vi "validate configuration.vi"(8 "error in":errorcluster, 11 "Profibus Module configuration in":refnum<class "Profibus Module configuration.lvclass">) -> (0 "error out":errorcluster, 3 "Profibus Module configuration out":refnum<class "Profibus Module configuration.lvclass">)   [LabVIEW 2013, in "Profibus Module configuration.lvclass"]
doc: "This function performs validation of the configuration. This function should be safe to call at any point and should not rely on anything in the runtime environment."
uses:
  Profibus Module configuration.lvclass
  <vilib>/NI/Tag Bus Module Framework/module configuration/TBM module configuration.lvclass
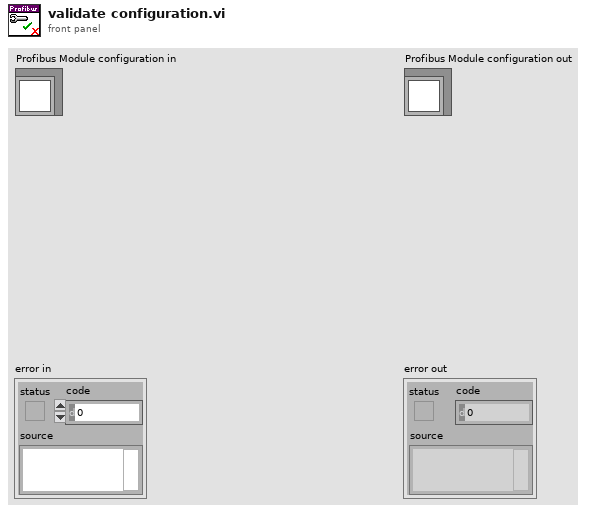
[diagram p1: front panel]
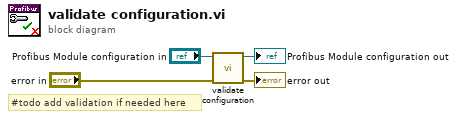
[diagram p0: block diagram]
diagram:
  # "#todo add validation if needed here"
  n1 = call-parent "validate configuration.vi"("error in"="error in", "configuration in"="Profibus Module configuration in") -> ("error out"=→"error out":errorcluster, "configuration out"=→"Profibus Module configuration out":refnum<class "Profibus Module configuration.lvclass">)  [unwired: 8 in]
